vi "DataToDisplay.vi"(8 "error in (no error)":errorcluster, 11 "SimpleAF in":refnum<class "Counter.lvclass">) -> (0 "error out":errorcluster, 3 "SimpleAF out":refnum<class "Counter.lvclass">)   [LabVIEW 2013, in "Counter.lvclass"]
uses:
  Counter.lvclass
  Counter.lvclass/Counter.ctl
  DisplayUI Messages/Updata Msg/Updata Msg.lvclass/Updata Msg.ctl
  <vilib>/ActorFramework/Message Enqueuer/Message Enqueuer.lvclass/Message Enqueuer.ctl
  <vilib>/ActorFramework/Message Enqueuer/Enqueue.vi
  <vilib>/ActorFramework/Message Priority Queue/Priority Enqueue.vi
  DisplayUI Messages/Updata Msg/Updata Msg.lvclass
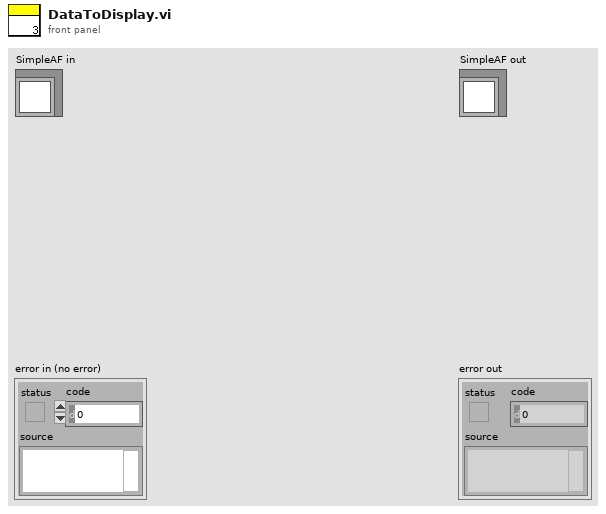
[diagram p1: front panel]
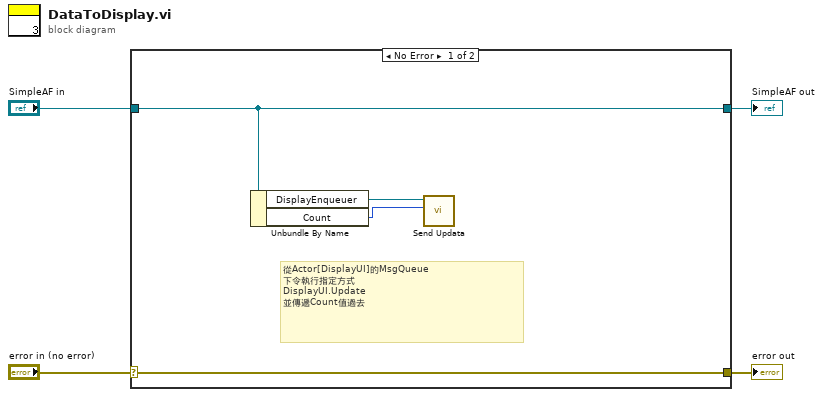
[diagram p0: block diagram]
diagram:
  n1 = case shown="No Error" "error in (no error)" {
    selector: "error in (no error)" -> [w8 w10]
    tunnel: [w8 w10] -> w3
    tunnel: [w7 w9] -> w1
    tunnel: "SimpleAF in" -> [w7 w9]
    frame No Error {
      # "從Actor[DisplayUI]的MsgQueue\n下令執行指定方式\nDisplayUI.Update\n並傳遞Count值過去"
      n2 = Unbundle By Name(w7) -> ("DisplayEnqueuer"=w5:refnum<class "Message Enqueuer.lvclass">, "Count"=w6:i32)
      n3 = call "Send Updata.vi"("Count"=w6, "Message Enqueuer"=w5) -> ()  [unwired: 8 in, 2 out]
    }
    frame Error {
    }
  }
  "error out" <- w3
  "SimpleAF out" <- w1
